vi "Set.vi"(6 "error":errorcluster, 7 "Input Command String":string, 8 "Quantity":string(combo), 9 "VISA resource name":refnum<visa-resource-name>) -> (0 "error out":errorcluster, 2 "Returned":dbl format="%_4f", 3 "VISA resource name out":refnum<visa-resource-name>, 5 "Response":string)   [LabVIEW 2018, in "BigSkyControl.lvlib"]
uses:
  BigSkyControl.lvlib
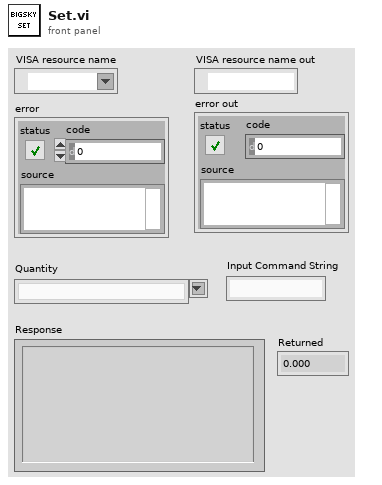
[diagram p1: front panel]
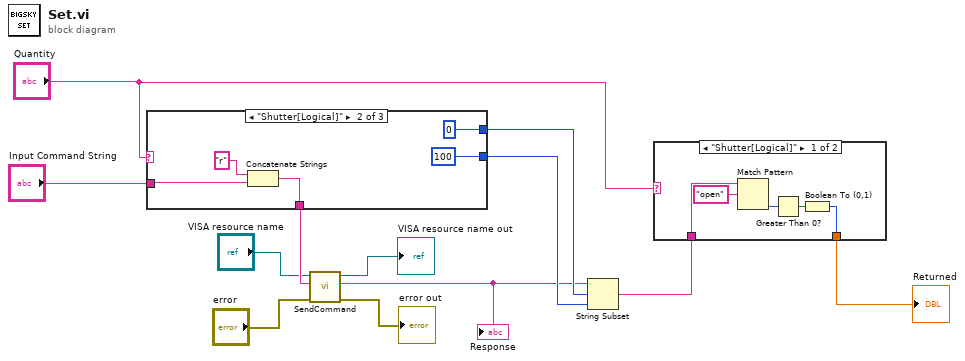
[diagram p0: block diagram]
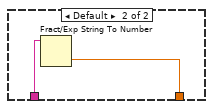
[diagram p2: hidden frame]
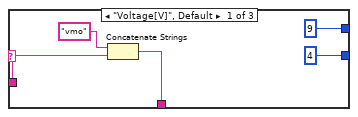
[diagram p3: hidden frame]
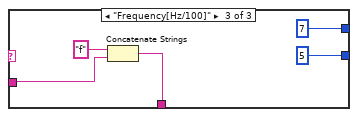
[diagram p4: hidden frame]
diagram:
  n1 = case shown="\"Shutter[Logical]\"" "Quantity" {
    tunnel: [w13 w18 w23] -> w6
    tunnel: [9 ("offset (0)") 0 ("offset (0)") 7 ("offset (0)")] -> w12
    tunnel: [4 ("length (rest)") 100 ("length (rest)") 5 ("length (rest)")] -> w11
    tunnel: "Input Command String" -> [w14 w19 w24]
    frame "Voltage[V]", Default {
      n2 = Concatenate Strings("vmo" ("string"), w14) -> (w13:string)
    }
    frame "Shutter[Logical]" {
      n3 = Concatenate Strings("r" ("string"), w19) -> (w18:string)
    }
    frame "Frequency[Hz/100]" {
      n4 = Concatenate Strings("f" ("string"), w24) -> (w23:string)
    }
  }
  n5 = call "SendCommand.vi"("error"="error", "write buffer (don't include >\\r\\n)"=w6, "VISA resource name"="VISA resource name") -> ("error out"=→"error out":errorcluster, "Response"=w1:string, "VISA resource name out"=→"VISA resource name out":refnum<visa-resource-name>)  [unwired: 6 in]
  "Response" <- w1
  n6 = String Subset(string=w1, offset (0)=w12, length (rest)=w11) -> (substring=w8:string)
  n7 = case shown="\"Shutter[Logical]\"" "Quantity" {
    tunnel: w8 -> [w32 w34]
    tunnel: [w28 w33] -> w7
    frame "Shutter[Logical]" {
      n8 = Match Pattern(string=w32, regular expression="open") -> (offset past match=w30:i32)  [unwired: 1 in, 3 out]
      n9 = Greater Than 0?(x=w30) -> (x > 0?=w29:bool)
      n10 = Boolean To (0,1)(Boolean=w29) -> (0, 1=w28:i16)
    }
    frame Default {
      n11 = Fract/Exp String To Number(string=w34) -> (number=w33:dbl)  [unwired: 3 in, 1 out]
    }
  }
  "Returned" <- w7
